vi "Unflatten UIP Value.vi"(10 "String Value":string, 11 "UIP In":refnum<class "TipStripUIP.lvclass">) -> (0 "Error Out":errorcluster, 3 "UIP Out":refnum<class "TipStripUIP.lvclass">)   [LabVIEW 2015, in "TipStripUIP.lvclass"]
uses:
  TipStripUIP.lvclass
  TipStripUIP.lvclass/TipStripUIP.ctl
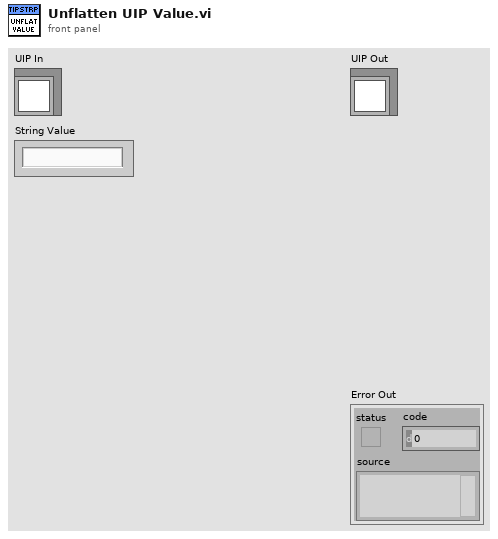
[diagram p1: front panel]
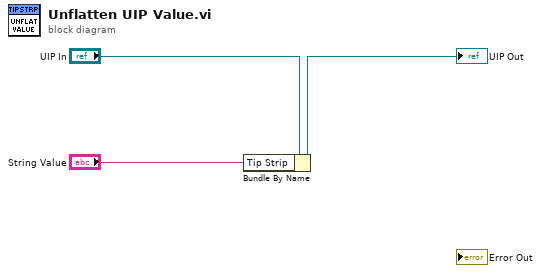
[diagram p0: block diagram]
diagram:
  n1 = Bundle By Name(cluster="UIP In", "Tip Strip"="String Value") -> (→"UIP Out":refnum<class "TipStripUIP.lvclass">)
